vi "auto mode control.vi"(0 "Pause":bool, 1 "Start":bool, 2 "Send GCode":bool, 5 "AUTO FR":i8, 7 "GCode":string, 9 "RESET":bool, 12 "Xs0":bool, 13 "Ys0":bool, 14 "Zs0":bool) -> (4 "Send command":string, 6 "Valid command":bool)   [LabVIEW 2014, in "HPCNC.lvlib"]
uses:
  HPCNC.lvlib
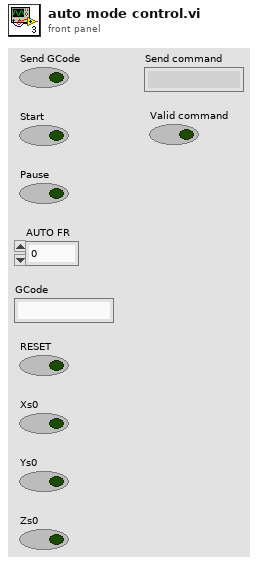
[diagram p1: front panel]
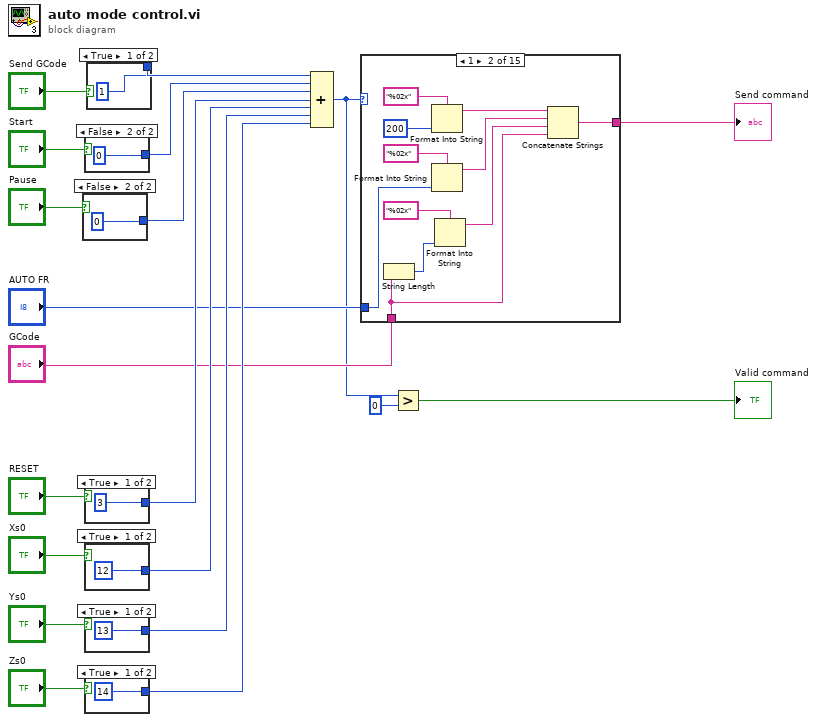
[diagram p0: block diagram]
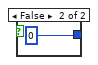
[diagram p2: hidden frame]
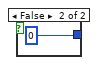
[diagram p3: hidden frame]
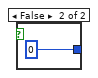
[diagram p4: hidden frame]
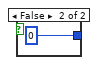
[diagram p5: hidden frame]
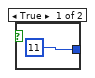
[diagram p6: hidden frame]
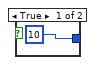
[diagram p7: hidden frame]
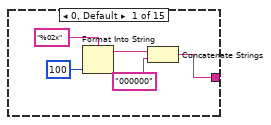
[diagram p8: hidden frame]
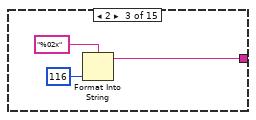
[diagram p9: hidden frame]
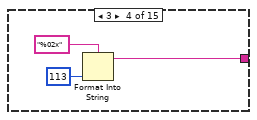
[diagram p10: hidden frame]
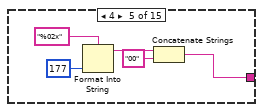
[diagram p11: hidden frame]
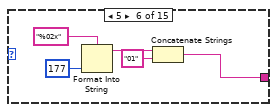
[diagram p12: hidden frame]
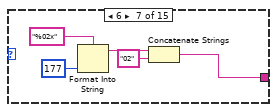
[diagram p13: hidden frame]
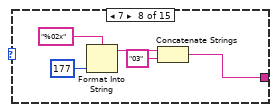
[diagram p14: hidden frame]
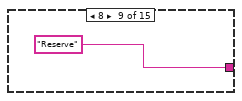
[diagram p15: hidden frame]
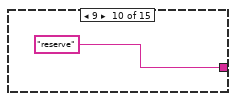
[diagram p16: hidden frame]
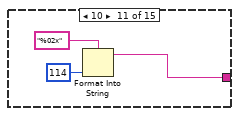
[diagram p17: hidden frame]
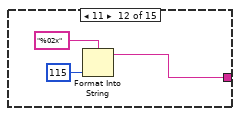
[diagram p18: hidden frame]
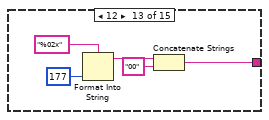
[diagram p19: hidden frame]
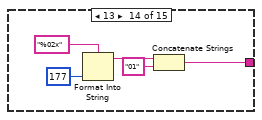
[diagram p20: hidden frame]
diagram:
  n1 = case shown="False" "Pause" {
    tunnel: [11 0] -> w7
    frame True {
    }
    frame False {
    }
  }
  n2 = case shown="False" "Start" {
    tunnel: [10 0] -> w6
    frame True {
    }
    frame False {
    }
  }
  n3 = case shown="True" "RESET" {
    tunnel: [3 0] -> w13
    frame True {
    }
    frame False {
    }
  }
  n4 = case shown="True" "Xs0" {
    tunnel: [12 0] -> w14
    frame True {
    }
    frame False {
    }
  }
  n5 = case shown="True" "Ys0" {
    tunnel: [13 0] -> w15
    frame True {
    }
    frame False {
    }
  }
  n6 = case shown="True" "Zs0" {
    tunnel: [14 0] -> w16
    frame True {
    }
    frame False {
    }
  }
  n7 = case shown="True" "Send GCode" {
    tunnel: [1 0] -> w1
    frame True {
    }
    frame False {
    }
  }
  n8 = Compound Arithmetic op=ADD(w1, w6, w7, w13, w14, w15, w16) -> (w2:i32)
  n9 = case shown="1" w2 {
    tunnel: [w35 w42 w51 w54 w57 w62 w67 w72 "Reserve" "reserve" w79 w82 w85 w90 w95] -> w5
    tunnel: "AUTO FR" -> [_ w41 _ _ _ _ _ _ _ _ _ _ _ _ _]
    tunnel: "GCode" -> [_ w40 _ _ _ _ _ _ _ _ _ _ _ _ _]
    frame 0, Default {
      n10 = Format Into String(format string="%02x", 100) -> (resulting string=w37:string)  [unwired: 2 in, 1 out]
      n11 = Concatenate Strings(w37, "000000" ("string")) -> (w35:string)
    }
    frame 1 {
      n12 = String Length(string=w40) -> (length=w44:i32)
      n13 = Format Into String(format string="%02x", 200) -> (resulting string=w48:string)  [unwired: 2 in, 1 out]
      n14 = Format Into String(format string="%02x", w41) -> (resulting string=w46:string)  [unwired: 2 in, 1 out]
      n15 = Format Into String(format string="%02x", w44) -> (resulting string=w43:string)  [unwired: 2 in, 1 out]
      n16 = Concatenate Strings(w48, w46, w43, w40) -> (w42:string)
    }
    frame 2 {
      n17 = Format Into String(format string="%02x", 116) -> (resulting string=w51:string)  [unwired: 2 in, 1 out]
    }
    frame 3 {
      n18 = Format Into String(format string="%02x", 113) -> (resulting string=w54:string)  [unwired: 2 in, 1 out]
    }
    frame 4 {
      n19 = Format Into String(format string="%02x", 177) -> (resulting string=w59:string)  [unwired: 2 in, 1 out]
      n20 = Concatenate Strings(w59, "00" ("string")) -> (w57:string)
    }
    frame 5 {
      n21 = Format Into String(format string="%02x", 177) -> (resulting string=w64:string)  [unwired: 2 in, 1 out]
      n22 = Concatenate Strings(w64, "01" ("string")) -> (w62:string)
    }
    frame 6 {
      n23 = Format Into String(format string="%02x", 177) -> (resulting string=w69:string)  [unwired: 2 in, 1 out]
      n24 = Concatenate Strings(w69, "02" ("string")) -> (w67:string)
    }
    frame 7 {
      n25 = Format Into String(format string="%02x", 177) -> (resulting string=w74:string)  [unwired: 2 in, 1 out]
      n26 = Concatenate Strings(w74, "03" ("string")) -> (w72:string)
    }
    frame 8 {
    }
    frame 9 {
    }
    frame 10 {
      n27 = Format Into String(format string="%02x", 114) -> (resulting string=w79:string)  [unwired: 2 in, 1 out]
    }
    frame 11 {
      n28 = Format Into String(format string="%02x", 115) -> (resulting string=w82:string)  [unwired: 2 in, 1 out]
    }
    frame 12 {
      n29 = Format Into String(format string="%02x", 177) -> (resulting string=w87:string)  [unwired: 2 in, 1 out]
      n30 = Concatenate Strings(w87, "00" ("string")) -> (w85:string)
    }
    frame 13 {
      n31 = Format Into String(format string="%02x", 177) -> (resulting string=w92:string)  [unwired: 2 in, 1 out]
      n32 = Concatenate Strings(w92, "01" ("string")) -> (w90:string)
    }
    frame 14 {
      n33 = Format Into String(format string="%02x", 177) -> (resulting string=w97:string)  [unwired: 2 in, 1 out]
      n34 = Concatenate Strings(w97, "02" ("string")) -> (w95:string)
    }
  }
  "Send command" <- w5
  n35 = Greater?(x=w2, y=0) -> (0:→"Valid command":bool)
